vi "niRFUtil WFM Decimate Waveform (real array).vi"(0 "Real Array In":T1 min=0 max=127 format="%.2f", 5 "Rate (1)":i32=1, 7 "Offset (0)":i32, 13 "Average? (F)":bool) -> (4 "Real Array Out":T1 min=0 max=127 format="%.2f")   [LabVIEW 2015, in "niRFUtil.lvlib"]
doc: "(c) Copyright 2006, National Instruments, Inc. This VI may not be duplicated, sold, or distributed without written consent from National Instruments."
uses:
  niRFUtil.lvlib
  Includes/niRFUtil INC Real Array.ctl
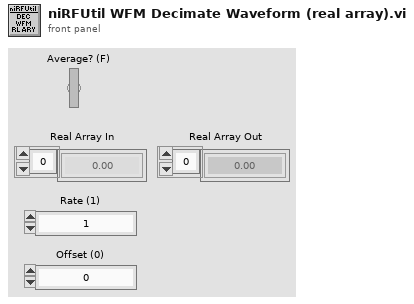
[diagram p1: front panel]
types:
  T1 = typedef "niRFUtil.lvlib/niRFUtil INC Real Array.ctl" = sgl[]
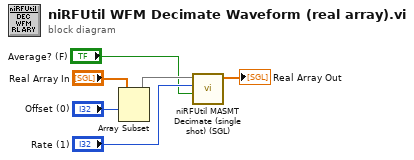
[diagram p0: block diagram]
diagram:
  n1 = Array Subset(array="Real Array In", index="Offset (0)") -> (w6:T1)  [unwired: 1 in]
  n2 = call "niRFUtil MASMT Decimate (single shot) (SGL).vi"("averaging"="Average? (F)", "decimating factor"="Rate (1)", "X"=w6) -> ("Decimated X"=→"Real Array Out":sgl[])  [unwired: 7 in, 1 out]
